vi "checkStatus.vi"(8 "error in (no error)":errorcluster, 10 "stop":bool, 11 "NetworkPixelfly in":refnum<class "Network_ProEm_WinX32.lvclass">) -> (0 "error out":errorcluster, 2 "stopped?":bool, 3 "NetworkPixelfly out":refnum<class "Network_ProEm_WinX32.lvclass">)   [LabVIEW 2011, in "Hardware.lvlib" / "HWControllers.lvlib" / "Network_ProEm_WinX32.lvclass"]
uses:
  Network_ProEm_WinX32.lvclass
  NetworkCamera.lvclass
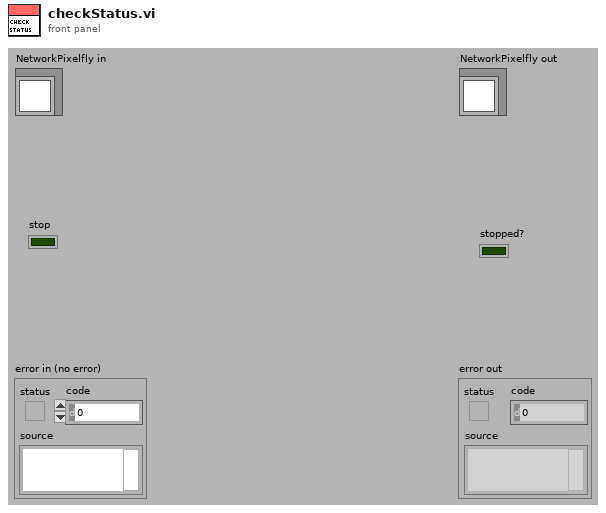
[diagram p1: front panel]
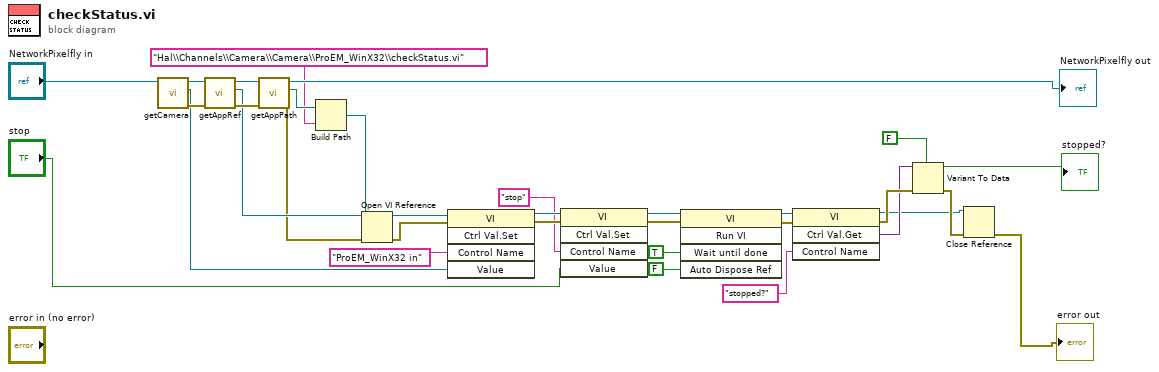
[diagram p0: block diagram]
diagram:
  n1 = call "getCamera.vi"("NetworkCamera in"="NetworkPixelfly in") -> ("error out"=w26:errorcluster, "Camera"=w17:refnum<class "Camera.lvclass">, "NetworkCamera out"=w28:refnum<class "Network_ProEm_WinX32.lvclass">)  [unwired: 8 in]
  n2 = call "getAppRef.vi"("error in (no error)"=w26, "NetworkCamera in"=w28) -> ("error out"=w25:errorcluster, "appRef"=w22:refnum<vi>, "NetworkCamera out"=w27:refnum<class "Network_ProEm_WinX32.lvclass">)  [unwired: 7 in]
  n3 = call "getAppPath.vi"("error in (no error)"=w25, "NetworkCamera in"=w27) -> ("error out"=w20:errorcluster, "appPath"=w24:path, "NetworkCamera out"=→"NetworkPixelfly out":refnum<class "Network_ProEm_WinX32.lvclass">)  [unwired: 7 in]
  n4 = Build Path(base path=w24, name or relative path="Hal\\Channels\\Camera\\Camera\\ProEM_WinX32\\checkStatus.vi") -> (appended path=w21:path)
  n5 = Open VI Reference(application reference (local)=w22, vi path=w21, error in (no error)=w20) -> (vi reference=w18:refnum<vi>, error out=w19:errorcluster)  [unwired: 3 in]
  n6 = invoke class="VI" method="Ctrl Val.Set"(reference=w18, error in=w19, "Control Name"="ProEM_WinX32 in", "Value"=w17) -> (reference out=w15:refnum<vi>, error out=w14:errorcluster)  [unwired: 1 in, 3 out]
  n7 = invoke class="VI" method="Ctrl Val.Set"(reference=w15, error in=w14, "Control Name"="stop", "Value"="stop") -> (reference out=w11:refnum<vi>, error out=w12:errorcluster)  [unwired: 1 in, 3 out]
  n8 = invoke class="VI" method="Run VI"(reference=w11, error in=w12, "Wait until done"=TRUE ("Wait Until Done"), "Auto Dispose Ref"=FALSE ("Auto Dispose Reference")) -> (reference out=w7:refnum<vi>, error out=w8:errorcluster)  [unwired: 1 in, 3 out]
  n9 = invoke class="VI" method="Ctrl Val.Get"(reference=w7, error in=w8, "Control Name"="stopped?") -> (reference out=w2:refnum<vi>, error out=w5:errorcluster, "Get Control Value Variant"=w4:variant)  [unwired: 1 in, 1 out]
  n10 = Variant To Data(error in=w5, type=FALSE, Variant=w4) -> (data=→"stopped?":bool, error out=w3:errorcluster)
  n11 = Close Reference(reference=w2, error in (no error)=w3) -> (error out=→"error out":errorcluster)
